vi "Set Sciscan Scope Focus.vi"(8 "error in":errorcluster, 10 "Focus Button":bool, 11 "GFG Refnum":refnum<vi>) -> (0 "error out":errorcluster, 3 "GFG Refnum Out":refnum<vi>)   [LabVIEW 2012, in "Sciscan Scope Daemon.lvlib"]
uses:
  Sciscan Scope Daemon.lvlib
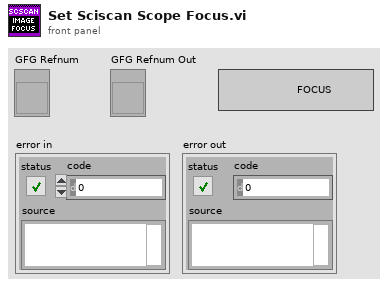
[diagram p1: front panel]
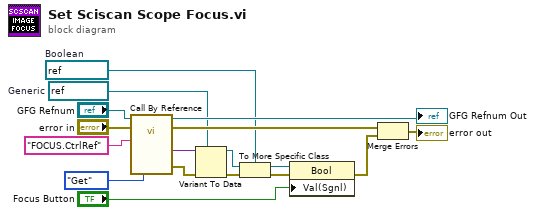
[diagram p0: block diagram]
diagram:
  w1 = refnum<vi> refnum  # Boolean
  w6 = refnum<vi> refnum  # Generic
  n1 = call-by-ref "?"(reference="GFG Refnum", error in="error in", "Variable Name in"="FOCUS.CtrlRef", "Action"=enum16{"Init", "Set", "Get"}."Get") -> (reference out=→"GFG Refnum Out":refnum<vi>, error out=w10:errorcluster, "Variant Out"=w14:variant, 19:"error out"=w11:errorcluster)  [unwired: 11 in, 5 out]
  n2 = Variant To Data(error in=w11, type=w6, Variant=w14) -> (data=w2:refnum<vi>, error out=w4:errorcluster)
  n3 = To More Specific Class(target class=w1, reference=w2, error in=w4) -> (specific class reference=w3:refnum<vi>, error out=w5:errorcluster)
  n4 = property class="Bool"(reference=w3, error in=w5, "Val(Sgnl)"="Focus Button") -> (error out=w9:errorcluster)  [unwired: 1 out]
  n5 = Merge Errors(w10, w9) -> (→"error out":errorcluster)
